vi "NI prepare task.vi"(8 "error in (no error)":errorcluster, 10 "NI task parameters":T1, 11 "NI in":refnum<class "NI.lvclass">) -> (0 "error out":errorcluster, 3 "NI out":refnum<class "NI.lvclass">)   [LabVIEW 2021, in "NI.lvlib" / "NI.lvclass"]
uses:
  NI.lvclass
  C:/Program Files (x86)/National Instruments/LabVIEW 2021/vi.lib/ActorFramework/Actor/Actor.lvclass
  NI task parameters.ctl
  NI.lvclass/NI.ctl
  Main_Control/Main_Control/notifications.ctl
  <vilib>/ActorFramework/Actor/Actor.lvclass/Actor.ctl
  Main_Control/Main_Control Messages/UI notifier Msg/UI notifier Msg.lvclass/UI notifier Msg.ctl
  <vilib>/ActorFramework/Message Enqueuer/Message Enqueuer.lvclass/Message Enqueuer.ctl
  <vilib>/ActorFramework/Message Enqueuer/Enqueue.vi
  Main_Control/Main_Control Messages/UI notifier Msg/UI notifier Msg.lvclass
  C:/Program Files (x86)/National Instruments/LabVIEW 2021/vi.lib/ActorFramework/Message/Message.lvclass
  <vilib>/ActorFramework/Message Priority Queue/Priority Enqueue.vi
  <vilib>/ActorFramework/Actor/Actor.lvclass
  Main_Control/Main_Control/Main_Control.lvclass
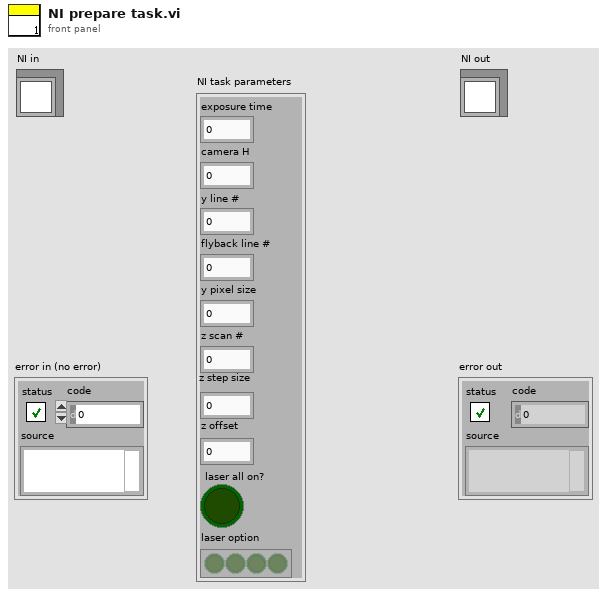
[diagram p1: front panel]
types:
  T1 = typedef "NI.lvlib/NI.lvclass/NI task parameters.ctl" = cluster{"exposure time":dbl, "camera H":dbl, "y line #":dbl, "flyback line #":dbl, "y pixel size":dbl, "z scan #":dbl, "z step size":dbl, "z offset":dbl, "laser all on?":bool, "laser option":bool[]}
  T2 = typedef "Main_Control.lvlib/Main_Control.lvclass/notifications.ctl" = enum16{"cam 1 frame skkipped", "cam finish", "cam started", "cam stopped", "cam updated", "ni started", "ni stopped", "ni updated"}
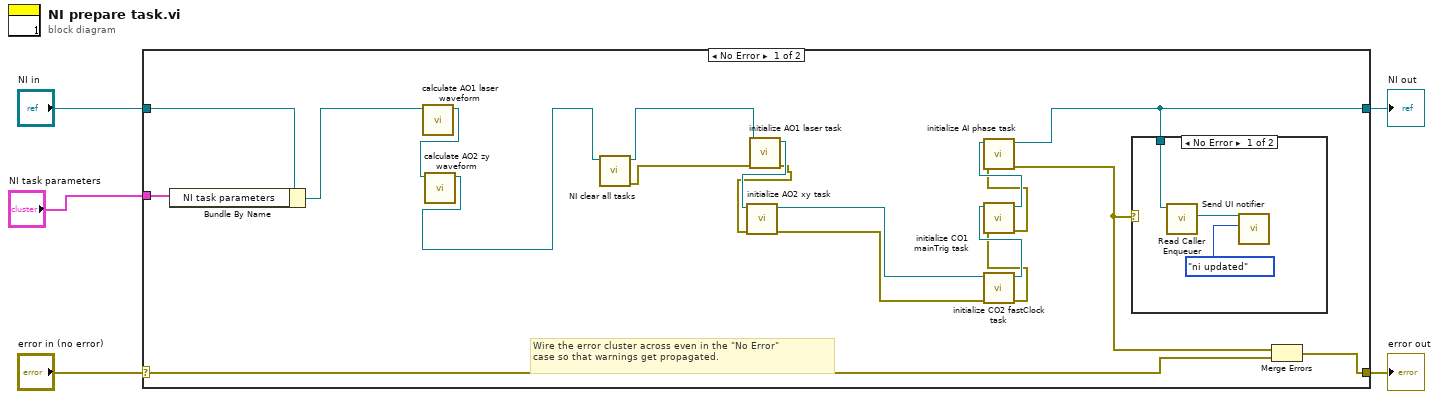
[diagram p0: block diagram]
diagram:
  n1 = case shown="No Error" "error in (no error)" {
    selector: "error in (no error)" -> [w13 w29]
    tunnel: [w12 w29] -> w4
    tunnel: [w10 w28] -> w2
    tunnel: "NI in" -> [w24 w28]
    tunnel: "NI task parameters" -> [w23 _]
    frame No Error {
      # "Wire the error cluster across even in the \"No Error\"\ncase so that warnings get propagated."
      n2 = Bundle By Name(cluster=w24, "NI task parameters"=w23) -> (w22:refnum<class "NI.lvclass">)
      n3 = call "calculate AO1 laser waveform.vi"("NI in"=w22) -> ("NI out"=w9:refnum<class "NI.lvclass">)  [unwired: 9 in, 1 out]
      n4 = call "calculate AO2 zy waveform.vi"("NI in"=w9) -> ("NI out"=w8:refnum<class "NI.lvclass">)  [unwired: 9 in, 1 out]
      n5 = call "NI clear all tasks.vi"("NI in"=w8) -> ("error out"=w17:errorcluster, "NI out"=w18:refnum<class "NI.lvclass">)  [unwired: 9 in]
      n6 = call "initialize AO1 laser task.vi"("error in (no error)"=w17, "NI in"=w18) -> ("error out"=w16:errorcluster, "NI out"=w21:refnum<class "NI.lvclass">)  [unwired: 8 in]
      n7 = call "initialize AO2 xy task.vi"("error in (no error)"=w16, "NI in"=w21) -> ("error out"=w6:errorcluster, "NI out"=w7:refnum<class "NI.lvclass">)  [unwired: 8 in]
      n8 = call "initialize CO2 fastClock task.vi"("error in (no error)"=w6, "NI in"=w7) -> ("error out"=w15:errorcluster, "NI out"=w20:refnum<class "NI.lvclass">)  [unwired: 8 in]
      n9 = call "initialize CO1 mainTrig task.vi"("error in (no error)"=w15, "NI in"=w20) -> ("error out"=w14:errorcluster, "NI out"=w19:refnum<class "NI.lvclass">)  [unwired: 8 in]
      n10 = call "initialize AI phase task.vi"("error in (no error)"=w14, "NI in"=w19) -> ("error out"=w11:errorcluster, "NI out"=w10:refnum<class "NI.lvclass">)  [unwired: 8 in]
      n11 = case shown="No Error" w11 {
        tunnel: w10 -> [w27 _]
        frame No Error {
          n12 = call <vilib>:"Read Caller Enqueuer.vi"("Actor"=w27) -> ("Caller Enqueuer"=w25:refnum<class "Message Enqueuer.lvclass">)  [unwired: 10 in]
          n13 = call "Send UI notifier.vi"("Object&State"=notifications."ni updated", "Message Enqueuer"=w25) -> ()  [unwired: 8 in, 2 out]
        }
        frame Error {
        }
      }
      n14 = Merge Errors(w11, w13) -> (w12:errorcluster)
    }
    frame Error {
    }
  }
  "error out" <- w4
  "NI out" <- w2
